vi "Sim status.vi"() -> ()   [LabVIEW 2014]
panel:
  out "Status":i32
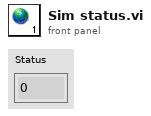
[diagram p1: front panel]
diagram:
